vi "PathDistance.vi"(10 "path":T1[](array[typedef])) -> (2 "distance":dbl)   [LabVIEW 2014, in "Waypoint.lvclass"]
uses:
  <userlib>/AdvancedDataStructures/ClassBased/Applications/RouteSearch/Waypoint/Waypoint.lvclass
  <userlib>/AdvancedDataStructures/ClassBased/Applications/RouteSearch/Waypoint/point.ctl
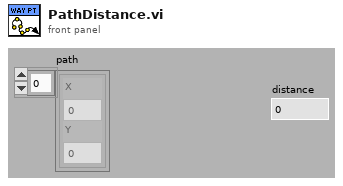
[diagram p1: front panel]
types:
  T1 = typedef "Waypoint.lvclass/point.ctl" = cluster{"X":dbl, "Y":dbl}
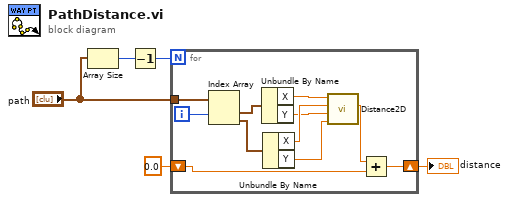
[diagram p0: block diagram]
diagram:
  n1 = Array Size(array="path") -> (size(s)=w3:i32)
  n2 = Decrement(x=w3) -> (x-1=w4:i32)
  n3 = for {
    N: w4 -> [_]
    tunnel: "path" -> [w16]
    shift-right: [w7] -> w1
    shift-left: 0.0 -> [w6]
    i -> [w15]
    n4 = Index Array(array=w16, index #1=w15) -> (element #1=w14:T1, element #2=w13:T1)  [unwired: 1 in]
    n5 = Unbundle By Name(w14) -> ("X"=w12:dbl, "Y"=w10:dbl)
    n6 = Unbundle By Name(w13) -> ("X"=w11:dbl, "Y"=w9:dbl)
    n7 = call <userlib>:"Distance2D.vi"("y2"=w9, "y1"=w10, "x2"=w11, "x1"=w12) -> ("distance"=w8:dbl)  [unwired: 7 in]
    n8 = Add(x=w8, y=w6) -> (x+y=w7:dbl)
  }
  "distance" <- w1
